vi "ADFX_Do_Save.vi"(8 "error in (no error)":errorcluster, 11 "Data in":T1) -> (0 "error out":errorcluster, 3 "Data out":T1)   [LabVIEW 2015]
doc: "Saves control data to file."
uses:
  controls/AFXP Data.ctl
  controls/AFCP Setup.ctl
  <vilib>/Utility/sysdir.llb/System Directory Type.ctl
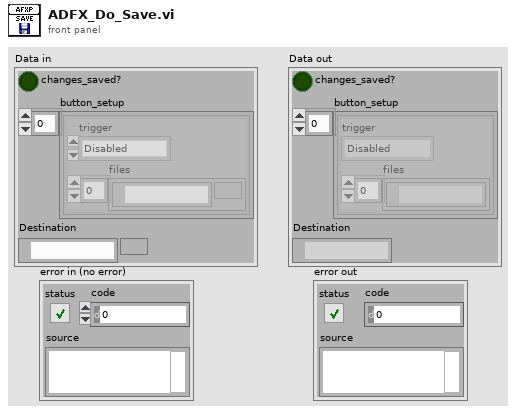
[diagram p1: front panel]
types:
  T1 = typedef "AFXP Data.ctl" = cluster{"changes_saved?":bool, "button_setup":T2[], "Destination":path}
  T2 = typedef "AFCP Setup.ctl" = cluster{"trigger":enum16{"Basic", "Hold-Loop", "Latch-Loop", "Next", "Random", "Disabled"}, "files":path[]}
  T3 = typedef "System Directory Type.ctl" = i32
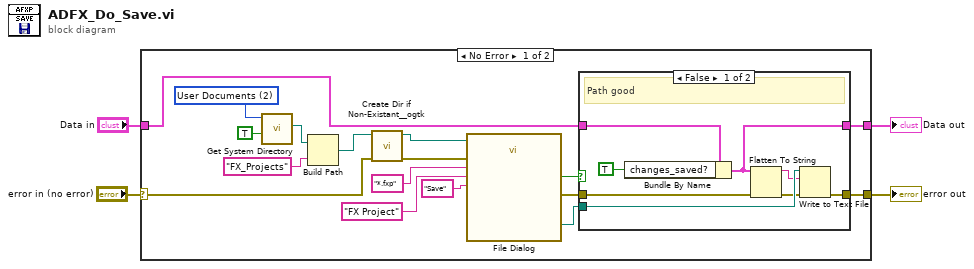
[diagram p0: block diagram]
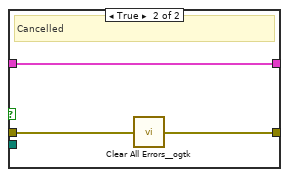
[diagram p2: hidden frame]
diagram:
  n1 = case shown="No Error" "error in (no error)" {
    selector: "error in (no error)" -> [w8 w33]
    tunnel: [w21 w34] -> w4
    tunnel: "Data in" -> [w7 w34]
    tunnel: [w10 w33] -> w2
    frame No Error {
      w5 = T3 2 items=["User Home"=0, "User Desktop"=1, "User Documents"=2, "User Application Data"=3, "User Preferences"=4, "User Temporary"=5, "Public Documents"=6, "Public Application Data"=7, "Public Preferences"=8, "Public Cache"=13, "System Core Libraries"=9, "System Installed Libraries"=10, "Application Files"=11, "Boot Volume Root"=12] ("system directory type")
      n2 = call <vilib>:"Get System Directory.vi"("create directory if not found? (F)"=TRUE, "system directory type"=w5) -> ("system directory"=w12:path)  [unwired: 9 in]
      n3 = Build Path(base path=w12, name or relative path="FX_Projects") -> (appended path=w19:path)
      n4 = call <userlib>:"Create Dir if Non-Existant__ogtk.vi"("error in (no error)"=w8, "Directory Path"=w19) -> ("error out"=w18:errorcluster, "dup Directory Path"=w20:path)  [unwired: 7 in, 1 out]
      n5 = call "File Dialog"("start path"=w20, "button label"="Save", "error in"=w18, "pattern (all files)"="*.fxp", "pattern label"="FX Project") -> ("selected path"=w11:path, "cancelled"=w17:bool, "error out"=w9:errorcluster)  [unwired: 7 in, 1 out]
      n6 = case shown="False" w17 {
        tunnel: w9 -> [w29 w32]
        tunnel: [w28 w30] -> w10
        tunnel: w11 -> [w27 _]
        tunnel: w7 -> [w24 w31]
        tunnel: [w22 w31] -> w21
        frame False {
          # "Path good"
          n7 = Bundle By Name(cluster=w24, "changes_saved?"=TRUE) -> (w22:T1)
          n8 = Flatten To String(anything=w22, error in (no error)=w29) -> (data string=w26:string, error out=w25:errorcluster)  [unwired: 2 in, 1 out]
          n9 = Write to Text File(file (use dialog)=w27, text=w26, error in=w25) -> (error out=w28:errorcluster)  [unwired: 1 in, 2 out]
        }
        frame True {
          # "Cancelled"
          n10 = call <userlib>:"Clear All Errors__ogtk.vi"("Error In"=w32) -> ("Error Out"=w30:errorcluster)  [unwired: 3 in]
        }
      }
    }
    frame Error {
    }
  }
  "Data out" <- w4
  "error out" <- w2
